vi "Digital Write.vi"   [LabVIEW 2018, in "LVH-LINX.lvlib"]
doc: "Write value(s) to the specified digital output channel(s)."
uses:
  LVH-LINX.lvlib
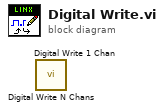
[diagram p0: block diagram]
diagram:
  n1 = call "Digital Write N Chans.vi"() -> ()  [unwired: 10 in, 2 out]
  n2 = call "Digital Write 1 Chan.vi"() -> ()  [unwired: 10 in, 2 out]
